vi "总磷总氮备用系数读取.vi"(8 "error in (no error)":errorcluster caption="错误输入（无错误）", 9 "量程":enum16{"低量程", "高量程"}(ring), 10 "测量模式":enum16{"水样测量", "空白核查", "跨度核查", "标样核查", "加标回收"}(ring), 11 "测量参数":enum16{"总磷", "总氮"}(ring)) -> (0 "error out":errorcluster caption="错误输出", 3 "备用系数":T1)   [LabVIEW 2016, in "斯坦道总氮.lvlib"]
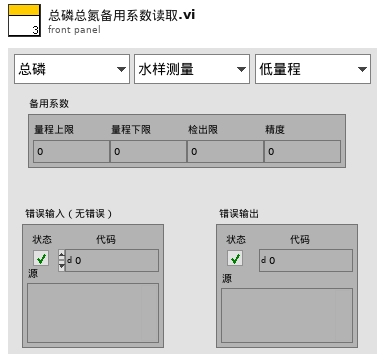
[diagram p1: front panel]
types:
  T1 = cluster{"量程上限":dbl, "量程下限":dbl, "检出限":dbl, "精度":dbl}
  T2 = cluster{"数组[0]":dbl, "数组[1]":dbl, "数组[2]":dbl, "数组[3]":dbl}
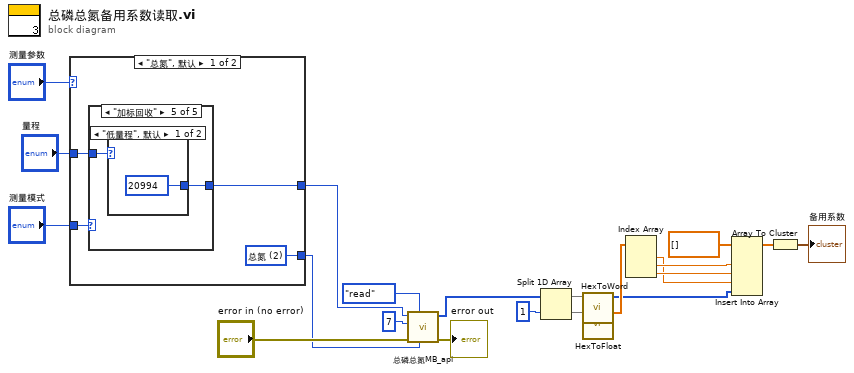
[diagram p0: block diagram]
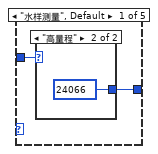
[diagram p2: hidden frame]
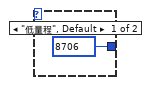
[diagram p3: hidden frame]
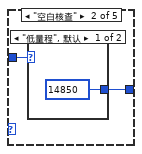
[diagram p4: hidden frame]
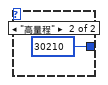
[diagram p5: hidden frame]
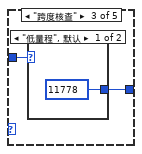
[diagram p6: hidden frame]
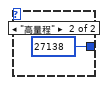
[diagram p7: hidden frame]
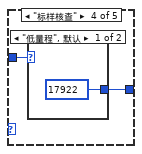
[diagram p8: hidden frame]
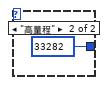
[diagram p9: hidden frame]
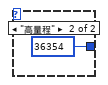
[diagram p10: hidden frame]
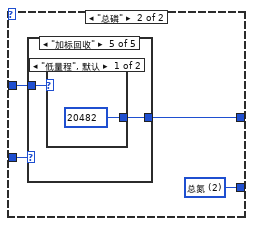
[diagram p11: hidden frame]
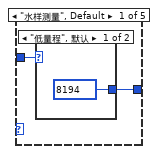
[diagram p12: hidden frame]
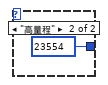
[diagram p13: hidden frame]
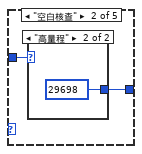
[diagram p14: hidden frame]
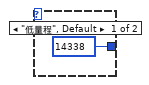
[diagram p15: hidden frame]
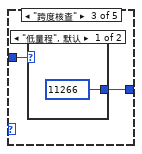
[diagram p16: hidden frame]
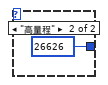
[diagram p17: hidden frame]
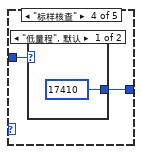
[diagram p18: hidden frame]
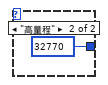
[diagram p19: hidden frame]
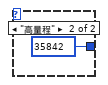
[diagram p20: hidden frame]
diagram:
  n1 = case shown="\"总氮\", 默认" "测量参数" {
    tunnel: "测量模式" -> [w25 w49]
    tunnel: "量程" -> [w24 w48]
    tunnel: [w23 w46] -> w1
    tunnel: [w22 w47] -> w2
    frame "总氮", Default {
      w23 = u16 2 items=["总磷"=1, "总氮"=2, "氨氮"=3] ("站号")
      n2 = case shown="\"加标回收\"" w25 {
        tunnel: w24 -> [w27 w31 w35 w39 w43]
        tunnel: [w26 w30 w34 w38 w42] -> w22
        frame "水样测量", Default {
          n3 = case shown="\"高量程\"" w27 {
            tunnel: [u16 8706 ("starting address") u16 24066 ("starting address")] -> w26
            frame "低量程", Default {
            }
            frame "高量程" {
            }
          }
        }
        frame "空白核查" {
          n4 = case shown="\"低量程\", 默认" w31 {
            tunnel: [u16 14850 ("starting address") u16 30210 ("starting address")] -> w30
            frame "低量程", Default {
            }
            frame "高量程" {
            }
          }
        }
        frame "跨度核查" {
          n5 = case shown="\"低量程\", 默认" w35 {
            tunnel: [u16 11778 ("starting address") u16 27138 ("starting address")] -> w34
            frame "低量程", Default {
            }
            frame "高量程" {
            }
          }
        }
        frame "标样核查" {
          n6 = case shown="\"低量程\", 默认" w39 {
            tunnel: [u16 17922 ("starting address") u16 33282 ("starting address")] -> w38
            frame "低量程", Default {
            }
            frame "高量程" {
            }
          }
        }
        frame "加标回收" {
          n7 = case shown="\"低量程\", 默认" w43 {
            tunnel: [u16 20994 ("starting address") u16 36354 ("starting address")] -> w42
            frame "低量程", Default {
            }
            frame "高量程" {
            }
          }
        }
      }
    }
    frame "总磷" {
      w46 = u16 2 items=["总磷"=1, "总氮"=2, "氨氮"=3] ("站号")
      n8 = case shown="\"加标回收\"" w49 {
        tunnel: w48 -> [w51 w55 w59 w63 w67]
        tunnel: [w50 w54 w58 w62 w66] -> w47
        frame "水样测量", Default {
          n9 = case shown="\"低量程\", 默认" w51 {
            tunnel: [u16 8194 ("starting address") u16 23554 ("starting address")] -> w50
            frame "低量程", Default {
            }
            frame "高量程" {
            }
          }
        }
        frame "空白核查" {
          n10 = case shown="\"高量程\"" w55 {
            tunnel: [u16 14338 ("starting address") u16 29698 ("starting address")] -> w54
            frame "低量程", Default {
            }
            frame "高量程" {
            }
          }
        }
        frame "跨度核查" {
          n11 = case shown="\"低量程\", 默认" w59 {
            tunnel: [u16 11266 ("starting address") u16 26626 ("starting address")] -> w58
            frame "低量程", Default {
            }
            frame "高量程" {
            }
          }
        }
        frame "标样核查" {
          n12 = case shown="\"低量程\", 默认" w63 {
            tunnel: [u16 17410 ("starting address") u16 32770 ("starting address")] -> w62
            frame "低量程", Default {
            }
            frame "高量程" {
            }
          }
        }
        frame "加标回收" {
          n13 = case shown="\"低量程\", 默认" w67 {
            tunnel: [u16 20482 ("starting address") u16 35842 ("starting address")] -> w66
            frame "低量程", Default {
            }
            frame "高量程" {
            }
          }
        }
      }
    }
  }
  n14 = call "总磷总氮MB_api.vi"("Slave ID"=w1, "STEP"=enum16{"open", "read", "write", "close"}."read", "Error in"="error in (no error)", "quantity"=u16 7, "starting address"=w2) -> ("error out"=→"error out":errorcluster, "Registers"=w18:u16[])  [unwired: 4 in, 1 out]
  n15 = Split 1D Array(array=w18, index=1 ("索引")) -> (first subarray=w16:u16[], second subarray=w15:u16[])
  n16 = call "HexToWord.vi"("数组"=w16) -> ("WORD"=w8:u16[])  [unwired: 10 in]
  n17 = call "HexToFloat.vi"("数组"=w15) -> ("FLOAT"=w13:sgl[])  [unwired: 10 in]
  n18 = Index Array(array=w13) -> (element #1=w9:sgl, element #2=w11:sgl, element #3=w10:sgl)  [unwired: 3 in]
  n19 = Insert Into Array(array=dbl[] [] ("数组"), new element #1=w11, new element #2=w10, new element #3=w9, new element #4=w8) -> (w7:dbl[])  [unwired: 1 in]
  n20 = Array To Cluster(array=w7) -> (cluster=→"备用系数":T2)
